vi "updateRate.vi"(10 "display rate":dbl=0.2 format="%#_13g", 11 "startTime":timestamp) -> (3 "Boolean":bool)   [LabVIEW 2016]
doc: "returns true if within 0.1 seconds of startTime+displayRate*n, where n is any whole number"
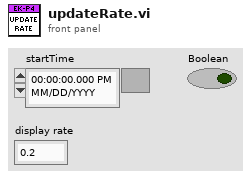
[diagram p1: front panel]
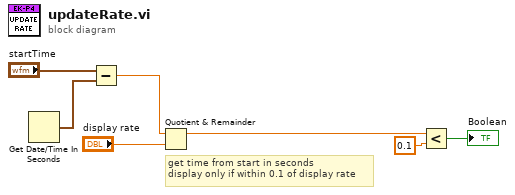
[diagram p0: block diagram]
diagram:
  # "get time from start in seconds\ndisplay only if within 0.1 of display rate"
  n1 = Get Date/Time In Seconds() -> (seconds since 1Jan1904=w1:timestamp)
  n2 = Subtract(x="startTime", y=w1) -> (x-y=w5:dbl)
  n3 = Quotient & Remainder(x=w5, y="display rate") -> (x-y*floor(x/y)=w7:dbl)  [unwired: 1 out]
  n4 = Less?(x=w7, y=0.1) -> (x < y?=→"Boolean":bool)
